vi "Decodificador_7seg.vi"() -> ()   [LabVIEW 2016]
panel:
  out "DISPLAY":T1
  in  "D":bool
  in  "C":bool
  in  "B":bool
  in  "A":bool
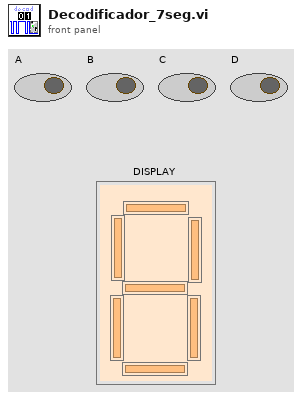
[diagram p1: front panel]
types:
  T1 = cluster{"SA":bool, "SB":bool, "SC":bool, "SD":bool, "SE":bool, "SF":bool, "SG":bool}
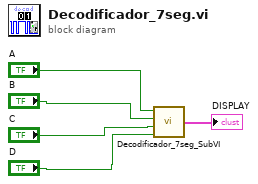
[diagram p0: block diagram]
diagram:
  n1 = call "Decodificador_7seg_SubVI.vi"("A"="D", "B"="C", "C"="B", "D"="A") -> ("DISPLAY"=→"DISPLAY":T1)
